vi "BRig_dataLC_init_setDefault.vi"(11 "input_dataLC":u16[](array[numeric])) -> (3 "output_dataLC":u16[](array[numeric]))   [LabVIEW 2014]
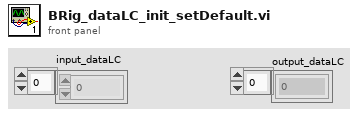
[diagram p1: front panel]
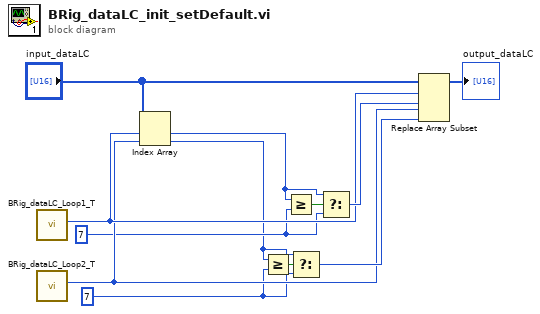
[diagram p0: block diagram]
diagram:
  w1 = u16 7 ("new element/subarray")
  w4 = u16 7 ("new element/subarray")
  n1 = call "BRig_dataLC_Loop1_T.vi"() -> ("output_Loop1_T"=w7:i32)  [unwired: 11 in]
  n2 = call "BRig_dataLC_Loop2_T.vi"() -> ("output_Loop2_T"=w6:i32)  [unwired: 11 in]
  n3 = Index Array(array="input_dataLC", index #1=w7, index #2=w6) -> (element #1=w5:u16, element #2=w2:u16)
  n4 = Greater Or Equal?(x=w2, y=w1) -> (x >= y?=w9:bool)
  n5 = Greater Or Equal?(x=w5, y=w4) -> (x >= y?=w3:bool)
  n6 = Select(t=w2, s=w9, f=w1) -> (s? t:f=w8:u16)
  n7 = Select(t=w5, s=w3, f=w4) -> (s? t:f=w10:u16)
  n8 = Replace Array Subset(array="input_dataLC", new element #1=w10, index #1=w7, new element #2=w8, index #2=w6) -> (→"output_dataLC":u16[])
